vi "Demo_CompressImageToMemory.vi"() -> ()   [LabVIEW 2024]
doc: "Compress into memory an image in any formats supported by QuickTime.\nUse QT_info.vi o learn about QT supported formats.\n\n© Ch. Salzmann, 1994-2003"
uses:
  <userlib>/ImageProcessing/QTLIB_2595_LV86/QT_Private.ctl
  <userlib>/ImageProcessing/QTLIB_2595_LV86/QT_Compression.ctl
  <userlib>/ImageProcessing/QTLIB_2595_LV86/QT_Image.ctl
panel:
  in  "Case Constant\n(See Context Help)":bool
  out "Image/Movie Out":T1 {"Dialogs" format="%.0b"}
  in  "Format":u16(ring)=1 items=["BMP", "JPEG", "MacPaint", "Photoshop", "PNG", "PICT", "QuickTime", "SG", "Targa", "TIFF"]
  in  "Compression":i32(slide)=498 scale=0.0..1023.0 scale format="%.0x"
  out "Image Source":picture
  out "error out":errorcluster
  # "Compress into memory an image in any formats\nsupported by QuickTime\n© Ch. Salzmann, 1994-2005"
  # "Min"
  # "Low"
  # "Normal"
  # "Hight"
  # "Max"
  # "Loss less"
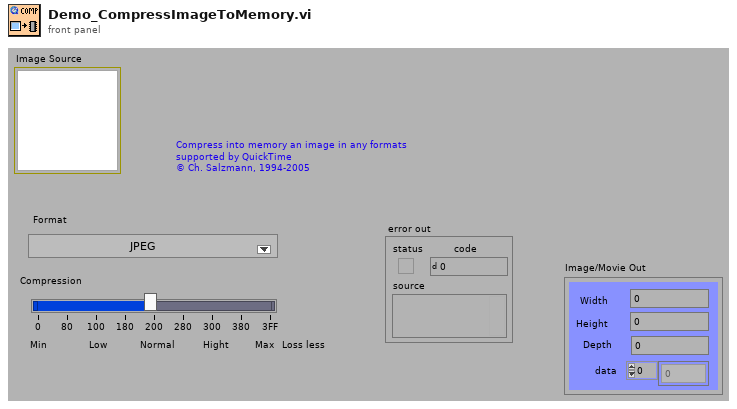
[diagram p1: front panel]
types:
  T1 = typedef "QT_Image.ctl" = cluster{"Width":i32, "Height":i32, "Depth":i32, "data":u8[], "Compressed data":u8[], "Color table":u32[], "Duration":i32, "Options":i32, "Timestamp":i32, "ID":i32, "Reserved":i32, "Dialogs":u32}
  T2 = typedef "QT_Compression.ctl" = cluster{"Compression":i32, "Format":i32, "Codec":i32, "Comp. Quality":i32, "Key Frame":i32, "Dialogs":u32}
  T3 = typedef "QT_Private.ctl" = cluster{"reserved 1":i32, "reserved 2":i32, "reserved 3":i32, "reserved 4":i32}
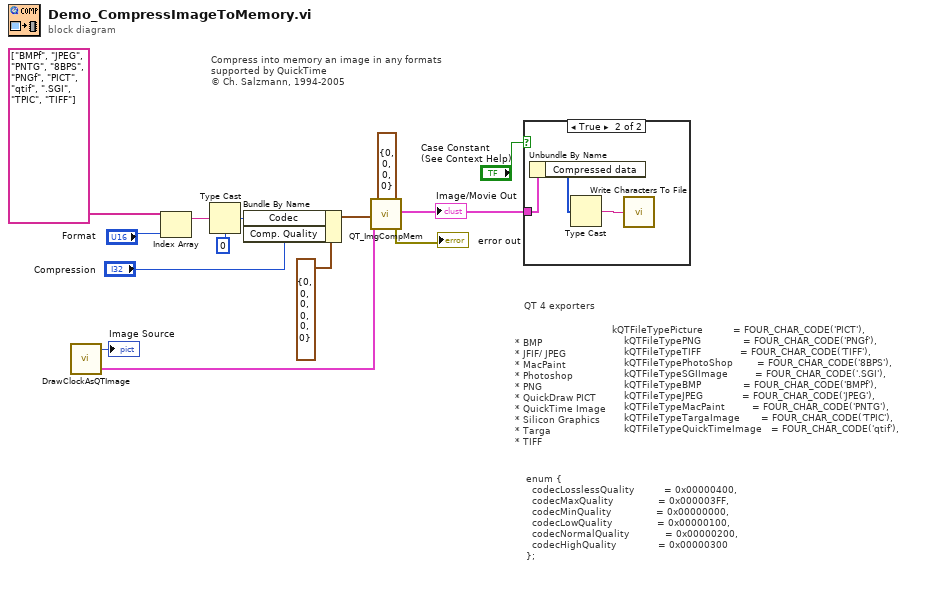
[diagram p0: block diagram]
diagram:
  # "QT 4 exporters"
  # "* BMP\n*\tJFIF/ JPEG \n*\tMacPaint\n*\tPhotoshop \n*\tPNG\n*\tQuickDraw PICT \n*\tQuickTime Image \n*\tSilicon Graphics\n*\tTarga\n*\tTIFF"
  # "kQTFileTypePicture          = FOUR_CHAR_CODE('PICT'),\n    kQTFileTypePNG              = FOUR_CHAR_CODE('PNGf'),\n    kQTFileTypeTIFF             = FOUR_CHAR_CODE('TIFF'),\n    kQTFileTypePhotoShop        = FOUR_CHAR_CODE('8BPS'),\n    kQTFileTypeSGIImage         = FOUR_CHAR_CODE('.SGI'),\n    kQTFileTypeBMP              = FOUR_CHAR_CODE('BMPf'),\n    kQTFileTypeJPEG             = FOUR_CHAR_CODE('JPEG'),\n    kQTFileTypeMacPaint         = FOUR_CHAR_CODE('PNTG'),\n    kQTFileTypeTargaImage       = FOUR_CHAR_CODE('TPIC'),\n    kQTFileTypeQuickTimeImage   = FOUR_CHAR_CODE('qtif'),"
  # "enum {\n  codecLosslessQuality          = 0x00000400,\n  codecMaxQuality               = 0x000003FF,\n  codecMinQuality               = 0x00000000,\n  codecLowQuality               = 0x00000100,\n  codecNormalQuality            = 0x00000200,\n  codecHighQuality              = 0x00000300\n};"
  # "Compress into memory an image in any formats\nsupported by QuickTime\n© Ch. Salzmann, 1994-2005"
  n1 = call <userlib>:"DrawClockAsQTImage.vi"() -> ("Picture"=→"Image Source":picture, "Image Out (24 bits)"=w10:T1)  [unwired: 2 in, 16 out]
  n2 = Index Array(array=string[] ["BMPf", "JPEG", "PNTG", "8BPS", "PNGf", "PICT", "qtif", ".SGI", "TPIC", "TIFF"], index="Format") -> (element=w5:string)
  n3 = Type Cast(type=0 ("Format"), x=w5) -> (*(type *) &x=w3:i32)
  n4 = Bundle By Name(cluster=T2 {"Compression"=0, "Format"=0, "Codec"=0, "Comp. Quality"=0, "Key Frame"=0, "Dialogs"=0} ("Compression Settings"), "Codec"=w3, "Comp. Quality"="Compression") -> (w13:T2)
  n5 = call <userlib>:"QT_ImgCompMem.vi"("Image In"=w10, "Compression Settings"=w13, "Private"=T3 {"reserved 1"=0, "reserved 2"=0, "reserved 3"=0, "reserved 4"=0}) -> ("Image/Movie Out"=w2:T1, "error out"=→"error out":errorcluster)  [unwired: 6 in, 9 out]
  "Image/Movie Out" <- w2
  n6 = case shown="True" "Case Constant\n(See Context Help)" {
    tunnel: w2 -> [_ w17]
    frame False {
    }
    frame True {
      n7 = Unbundle By Name(w17) -> ("Compressed data"=w16:u8[])
      n8 = Type Cast(x=w16) -> (*(type *) &x=w15:string)  [unwired: 1 out]
      n9 = call <vilib>:"Write Characters To File.vi"("character string"=w15) -> ()  [unwired: 2 in, 3 out]
    }
  }
